vi "32 BIT ONLY  - - - - robo move.vi"() -> ()   [LabVIEW 2026]
uses:
  <vilib>/ImagingLab/Denso Robotics Library/_Private/Controls/drl_Robot Coordinates.ctl
  <vilib>/ImagingLab/Denso Robotics Library/_Private/Controls/drl_Robot Session.ctl
  <vilib>/ImagingLab/Denso Robotics Library/_Private/Controls/drl_Open Data.ctl
  <vilib>/ImagingLab/Denso Robotics Library/_Private/Controls/drl_Controller_IP Address.ctl
  <vilib>/ImagingLab/Denso Robotics Library/_Private/Controls/drl_Robot type.ctl
  <vilib>/ImagingLab/Denso Robotics Library/_Private/Controls/drl_controller_type.ctl
  <vilib>/ImagingLab/Denso Robotics Library/_Private/Controls/drl_RobSlave actions.ctl
  <vilib>/ImagingLab/Denso Robotics Library/_Private/Controls/drl_Get_Set.ctl
  <vilib>/ImagingLab/Denso Robotics Library/_Private/Controls/drl_Robot Motor status.ctl
  <vilib>/ImagingLab/Denso Robotics Library/_Private/Controls/drl_Motion parameters.ctl
  <vilib>/ImagingLab/Denso Robotics Library/_Private/Controls/drl_Interpolation.ctl
  <vilib>/ImagingLab/Denso Robotics Library/_Private/Controls/drl_Pass motion.ctl
  <vilib>/ImagingLab/Denso Robotics Library/_Private/Controls/drl_Move option.ctl
  <vilib>/ImagingLab/Denso Robotics Library/_Public/SubVIs/drl_Robot Move_CARTESIAN.vi
  <vilib>/ImagingLab/Denso Robotics Library/_Public/SubVIs/drl_Get_Robot Position_P.vi
  <vilib>/ImagingLab/Denso Robotics Library/DensoRoboticsLibrary.lvlib
panel:
  out "cRIO RT Data":cluster{u16, u16, u16}
  in  "index":i32
  out "error out":errorcluster
  in  "stop":bool
  out "Robot Position":T1 {"X" format="%.4f"; "Y" format="%.4f"; "Z" format="%.4f"; "Rx" format="%.4f"; "Ry" format="%.4f"; "Rz" format="%.4f"}
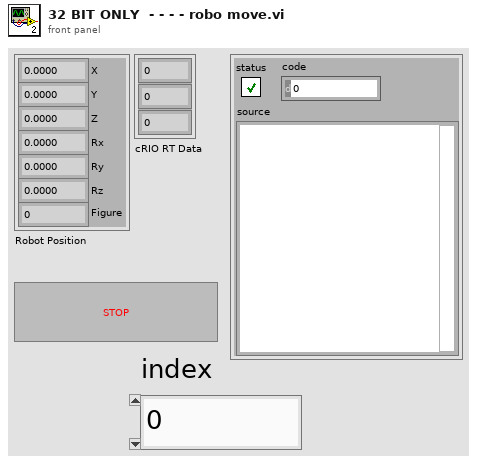
[diagram p1: front panel]
types:
  T1 = typedef "DensoRoboticsLibrary.lvlib/drl_Robot Coordinates.ctl" = cluster{"X":dbl, "Y":dbl, "Z":dbl, "Rx":dbl, "Ry":dbl, "Rz":dbl, "Figure":dbl}
  T2 = cluster{"X":dbl, "Y":dbl, "Z":dbl, "Rx":dbl, "Ry":dbl, "Rz":dbl, "Figure":dbl}
  T3 = typedef "DensoRoboticsLibrary.lvlib/drl_Motion parameters.ctl" = cluster{"Interpolation":T4, "Pass motion":T5, "Option":T6}
  T4 = typedef "DensoRoboticsLibrary.lvlib/drl_Interpolation.ctl" = enum16{"Move P", "Move L"}
  T5 = typedef "DensoRoboticsLibrary.lvlib/drl_Pass motion.ctl" = enum16{"@0", "@P", "@E"}
  T6 = typedef "DensoRoboticsLibrary.lvlib/drl_Move option.ctl" = enum16{"Default", "Next"}
  T7 = typedef "DensoRoboticsLibrary.lvlib/drl_Robot Motor status.ctl" = enum16{"Motor OFF", "Motor ON"}
  T8 = typedef "DensoRoboticsLibrary.lvlib/drl_Get_Set.ctl" = enum16{"Get", "Set"}
  T9 = typedef "DensoRoboticsLibrary.lvlib/drl_RobSlave actions.ctl" = enum16{"Start", "Stop"}
  T10 = typedef "DensoRoboticsLibrary.lvlib/drl_Open Data.ctl" = cluster{"controller IP address":T11, "robot type":T12, "controller type":T13}
  T11 = typedef "DensoRoboticsLibrary.lvlib/drl_Controller_IP Address.ctl" = string
  T12 = typedef "DensoRoboticsLibrary.lvlib/drl_Robot type.ctl" = enum16{"6 axes", "5 axes", "4 axes"}
  T13 = typedef "DensoRoboticsLibrary.lvlib/drl_controller_type.ctl" = enum16{"RC7", "RC8"}
  T14 = typedef "DensoRoboticsLibrary.lvlib/drl_Robot Session.ctl" = string
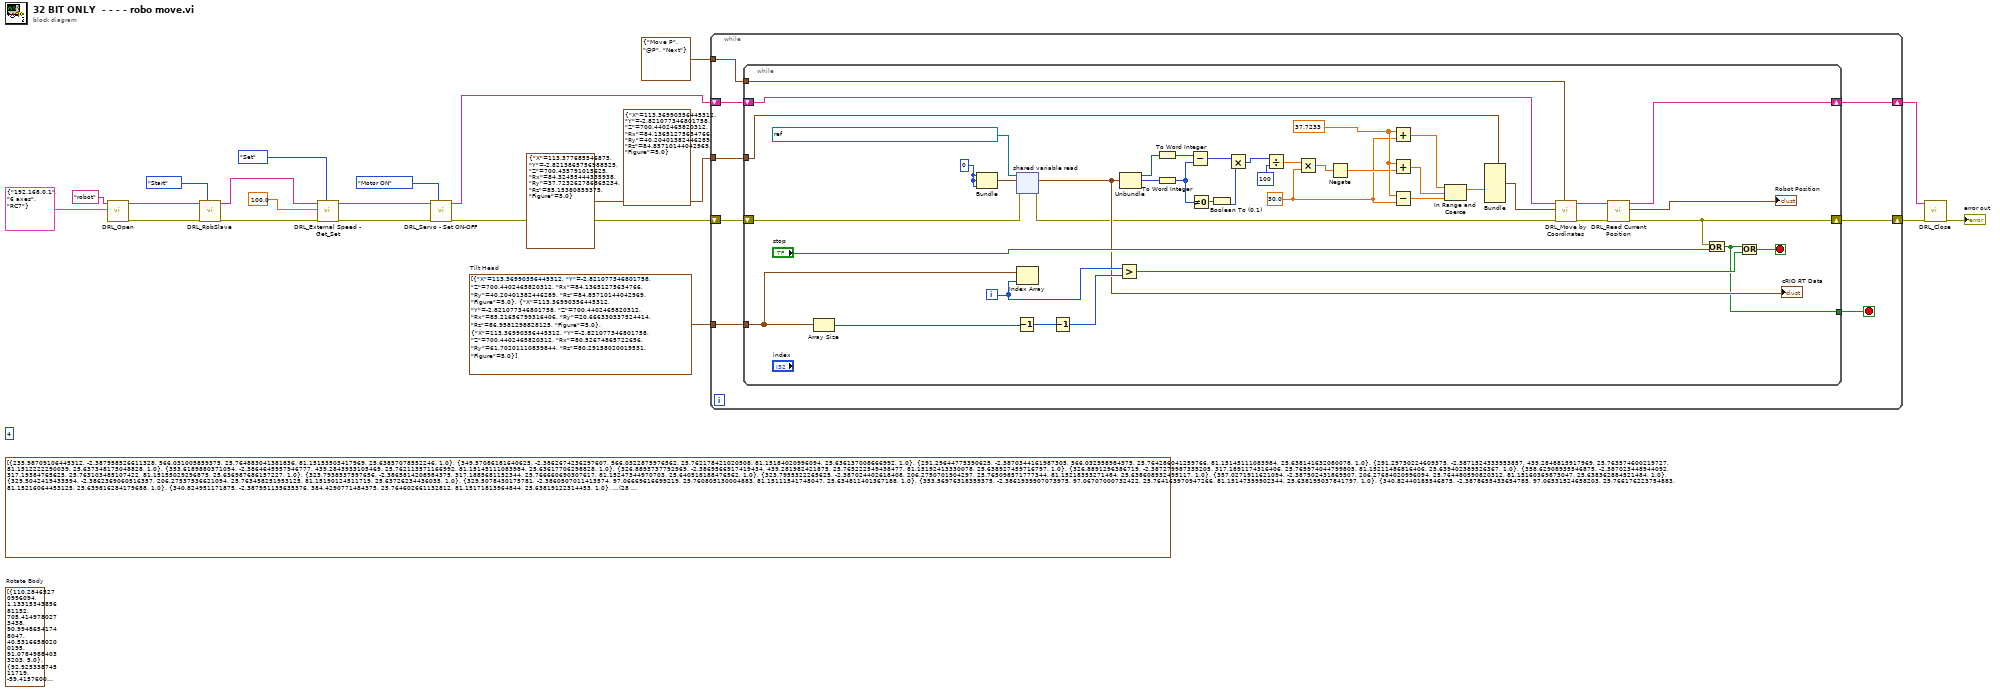
[diagram p0: block diagram]
diagram:
  (unwired) T1 {"X"=113.36990356445312, "Y"=-2.821077346801758, "Z"=700.4402465820312, "Rx"=84.13651275634766, "Ry"=40.20401382446289, "Rz"=84.85710144042969, "Figure"=5.0} ("position P")
  w2 = T1[] [{"X"=113.36990356445312, "Y"=-2.821077346801758, "Z"=700.4402465820312, "Rx"=84.13651275634766, "Ry"=40.20401382446289, "Rz"=84.85710144042969, "Figure"=5.0}, {"X"=113.36990356445312, "Y"=-2.821077346801758, "Z"=700.4402465820312, "Rx"=85.21656799316406, "Ry"=20.666330337524414, "Rz"=86.9581298828125, "Figure"=5.0}, {"X"=113.36990356445312, "Y"=-2.821077346801758, "Z"=700.4402465820312, "Rx"=80.52674865722656, "Ry"=61.70201110839844, "Rz"=80.29158020019531, "Figure"=5.0}]  # Tilt Head
  (unwired) T1[] [{"X"=110.28465270996094, "Y"=1.1331534385681152, "Z"=705.4149780273438, "Rx"=90.99486541748047, "Ry"=40.53166580200195, "Rz"=91.07849884033203, "Figure"=5.0}, {"X"=92.92533874511719, "Y"=-59.4157600402832, "Z"=705.412109375, "Rx"=90.99667358398438, "Ry"=40.53141784667969, "Rz"=57.89656448364258, "Figure"=5.0}, {"X"=90.63916778564453, "Y"=62.848175048828125, "Z"=705.412109375, "Rx"=90.99667358398438, "Ry"=40.53141784667969, "Rz"=125.22810363769531, "Figure"=5.0}]  # Rotate Body
  (unwired) T1[] [{"X"=235.98709106445312, "Y"=-2.387958526611328, "Z"=566.031005859375, "Rx"=25.764883041381836, "Ry"=81.15153503417969, "Rz"=25.63857078552246, "Figure"=1.0}, {"X"=349.57086181640625, "Y"=-2.3862674236297607, "Z"=566.0322875976562, "Rx"=25.762178421020508, "Ry"=81.15184020996094, "Rz"=25.636137008666992, "Figure"=1.0}, {"X"=291.29644775390625, "Y"=-2.3870344161987305, "Z"=566.032958984375, "Rx"=25.764286041259766, "Ry"=81.15145111083984, "Rz"=25.638141632080078, "Figure"=1.0}, {"X"=291.29730224609375, "Y"=-2.3871524333953857, "Z"=439.2848815917969, "Rx"=25.763574600219727, "Ry"=81.1512222290039, "Rz"=25.637348175048828, "Figure"=1.0}, {"X"=353.6189880371094, "Y"=-2.3864645957946777, "Z"=439.2843933105469, "Rx"=25.762113571166992, "Ry"=81.15145111083984, "Rz"=25.63617706298828, "Figure"=1.0}, {"X"=326.8893737792969, "Y"=-2.3869566917419434, "Z"=439.281982421875, "Rx"=25.765222549438477, "Ry"=81.15192413330078, "Rz"=25.638927459716797, "Figure"=1.0}, {"X"=326.8891296386719, "Y"=-2.387279987335205, "Z"=317.1891174316406, "Rx"=25.765974044799805, "Ry"=81.15211486816406, "Rz"=25.639402389526367, "Figure"=1.0}, {"X"=358.62908935546875, "Y"=-2.387023448944092, "Z"=317.19384765625, "Rx"=25.763103485107422, "Ry"=81.15155029296875, "Rz"=25.636987686157227, "Figure"=1.0}, {"X"=323.7938537597656, "Y"=-2.3865814208984375, "Z"=317.1885681152344, "Rx"=25.766660690307617, "Ry"=81.15247344970703, "Rz"=25.640518188476562, "Figure"=1.0}, {"X"=323.7955322265625, "Y"=-2.387024402618408, "Z"=206.2750701904297, "Rx"=25.765098571777344, "Ry"=81.15218353271484, "Rz"=25.638608932495117, "Figure"=1.0}, {"X"=357.0271911621094, "Y"=-2.387502431869507, "Z"=206.27684020996094, "Rx"=25.764480590820312, "Ry"=81.15160369873047, "Rz"=25.638362884521484, "Figure"=1.0}, {"X"=329.5042419433594, "Y"=-2.3862369060516357, "Z"=206.27537536621094, "Rx"=25.763458251953125, "Ry"=81.15190124511719, "Rz"=25.63726234436035, "Figure"=1.0}, {"X"=329.5078430175781, "Y"=-2.3860507011413574, "Z"=97.06669616699219, "Rx"=25.760805130004883, "Ry"=81.15111541748047, "Rz"=25.634811401367188, "Figure"=1.0}, {"X"=353.56976318359375, "Y"=-2.3861939907073975, "Z"=97.06707000732422, "Rx"=25.764163970947266, "Ry"=81.15147399902344, "Rz"=25.638195037841797, "Figure"=1.0}, {"X"=340.82440185546875, "Y"=-2.3878655433654785, "Z"=97.06531524658203, "Rx"=25.766176223754883, "Ry"=81.15216064453125, "Rz"=25.639816284179688, "Figure"=1.0}, {"X"=340.824951171875, "Y"=-2.387951135635376, "Z"=384.4290771484375, "Rx"=25.764602661132812, "Ry"=81.15171813964844, "Rz"=25.63819122314453, "Figure"=1.0}, {"X"=1.4659475088119507, "Y"=-340.9820861816406, "Z"=384.4298400878906, "Rx"=25.765399932861328, "Ry"=81.15129089355469, "Rz"=-63.7135124206543, "Figure"=1.0}, {"X"=1.4659475088119507, "Y"=-340.9820861816406, "Z"=384.4298400878906, "Rx"=25.765399932861328, "Ry"=81.15129089355469, "Rz"=-63.7135124206543, "Figure"=1.0}, {"X"=1.4495900869369507, "Y"=-336.9073791503906, "Z"=400.07806396484375, "Rx"=9.859703063964844, "Ry"=68.43805694580078, "Rz"=-79.16173553466797, "Figure"=1.0}, {"X"=1.449590802192688, "Y"=-336.9075927734375, "Z"=400.07757568359375, "Rx"=9.859916687011719, "Ry"=68.43849182128906, "Rz"=-79.16153717041016, "Figure"=1.0}, {"X"=1.4632148742675781, "Y"=-340.8019714355469, "Z"=363.8247375488281, "Rx"=156.8294677734375, "Ry"=80.24137878417969, "Rz"=66.77577209472656, "Figure"=1.0}, {"X"=1.4495900869369507, "Y"=-336.9073791503906, "Z"=400.07806396484375, "Rx"=9.859703063964844, "Ry"=68.43805694580078, "Rz"=-79.16173553466797, "Figure"=1.0}, {"X"=1.4632148742675781, "Y"=-340.8019714355469, "Z"=363.8247375488281, "Rx"=156.8294677734375, "Ry"=80.24137878417969, "Rz"=66.77577209472656, "Figure"=1.0}, {"X"=1.4669764041900635, "Y"=-341.2671813964844, "Z"=382.1100769042969, "Rx"=32.499534606933594, "Ry"=82.82139587402344, "Rz"=-57.044464111328125, "Figure"=1.0}, {"X"=340.9021301269531, "Y"=-15.848700523376465, "Z"=382.1100769042969, "Rx"=32.49953079223633, "Ry"=82.82139587402344, "Rz"=30.047452926635742, "Figure"=1.0}, {"X"=340.9021301269531, "Y"=-15.848700523376465, "Z"=382.1100769042969, "Rx"=32.49953079223633, "Ry"=82.82139587402344, "Rz"=30.047452926635742, "Figure"=1.0}, {"X"=340.9021301269531, "Y"=-15.848700523376465, "Z"=382.1100769042969, "Rx"=32.49953079223633, "Ry"=82.82139587402344, "Rz"=30.047452926635742, "Figure"=1.0}, {"X"=340.9021301269531, "Y"=-15.848700523376465, "Z"=382.1100769042969, "Rx"=32.49953079223633, "Ry"=82.82139587402344, "Rz"=30.047452926635742, "Figure"=1.0}] ("appended array")
  (unwired) 4
  n1 = call <vilib>:"DRL_Open.vi"("connection settings"=T10 {"controller IP address"="192.168.0.1", "robot type"=enum."6 axes", "controller type"=enum."RC7"}, "robot session"=T14 "robot") -> ("error out"=w6:errorcluster, "robot session*"=w7:T14)  [unwired: 8 in]
  n2 = call <vilib>:"DRL_RobSlave.vi"("action"=drl_RobSlave_actions."Start" ("Action"), "error in (no error)"=w6, "robot session"=w7) -> ("error out"=w8:errorcluster, "robot session*"=w9:T14)  [unwired: 7 out]
  n3 = call <vilib>:"DRL_External Speed - Get_Set.vi"("action"=drl_Get_Set."Set" ("Get / Set"), "error in (no error)"=w8, "ext speed in"=sgl 100.0 ("Ext Speed in"), "robot session"=w9) -> ("error out"=w11:errorcluster, "robot session*"=w10:T14)  [unwired: 6 out]
  n4 = call <vilib>:"DRL_Servo - Set ON-OFF.vi"("servo status"=drl_Robot_Motor_status."Motor ON" ("Motor Status"), "error in (no error)"=w11, "robot session"=w10) -> ("error out"=w4:errorcluster, "robot session*"=w5:T14)  [unwired: 7 out]
  n5 = while {
    tunnel: T3 {"Interpolation"=enum."Move P", "Pass motion"=enum."@P", "Option"=enum."Next"} ("motion parameters") -> [w24]
    shift-right: [w27] -> w17
    shift-left: w5 -> [w26]
    shift-right: [w28] -> w18
    shift-left: w4 -> [w25]
    tunnel: w2 -> [w23]
    tunnel: T2 {"X"=113.377685546875, "Y"=-2.8213865756988525, "Z"=700.435791015625, "Rx"=84.32455444335938, "Ry"=37.723262786865234, "Rz"=85.15380859375, "Figure"=5.0} -> [w21]
    stop <- w22 stop-if-true
    n6 = while {
      shift-right: [w68] -> w28
      shift-left: w25 -> [w30]
      shift-right: [w70] -> w27
      shift-left: w26 -> [w67]
      tunnel: w24 -> [w64]
      tunnel: w23 -> [w57]
      tunnel: [w35] -> w22
      tunnel: w21 -> [w55]
      i -> [w63]
      stop <- w61 stop-if-true
      w40 = 37.7233 ("y")
      w38 = 30.0 ("y")
      w52 = u16 0
      n7 = Array Size(array=w57) -> (size(s)=w62:i32)
      n8 = Bundle(w52, w52, w52) -> (w53:cluster{u16, u16, u16})  [unwired: 1 in]
      n9 = Decrement(x=w62) -> (x-1=w58:i32)
      n10 = shared-variable-read(refnum<k21> "ni.var.psp://SpeedOfVIght/RT ShardVariables/Final Score" ("shared variable refnum in"), w30, w53) -> (w29:errorcluster, w50:cluster{u16, u16, u16})  [unwired: 2 out]
      "cRIO RT Data" <- w50
      n11 = Index Array(array=w57, index=w63) -> ()  [unwired: 1 out]
      n12 = Decrement(x=w58) -> (x-1=w59:i32)
      n13 = Greater?(x=w63, y=w59) -> (0:w60:bool)
      n14 = Unbundle(w50) -> (w49:u16, w48:u16)  [unwired: 1 out]
      n15 = To Word Integer(number=w49) -> (16bit integer=w41:i16)
      n16 = To Word Integer(number=w48) -> (16bit integer=w34:i16)
      n17 = Subtract(x=w41, y=w34) -> (x-y=w47:i16)
      n18 = Not Equal To 0?(x=w34) -> (x != 0?=w33:bool)
      n19 = Boolean To (0,1)(Boolean=w33) -> (0, 1=w31:i16)
      n20 = Multiply(x=w47, y=w31) -> (x*y=w32:i16)
      n21 = Divide(x=w32, y=u16 100) -> (x/y=w45:dbl)
      n22 = Multiply(x=w45, y=w38) -> (x*y=w44:dbl)
      n23 = Negate(x=w44) -> (-x=w39:dbl)
      n24 = Add(x=w40, y=w38) -> (x+y=w37:dbl)
      n25 = Add(x=w40, y=w39) -> (x+y=w43:dbl)
      n26 = Subtract(x=w40, y=w38) -> (x-y=w36:dbl)
      n27 = In Range and Coerce(upper limit=w37, x=w43, lower limit=w36) -> (coerced(x)=w54:dbl)  [unwired: 1 out]
      n28 = Bundle(cluster=w55, "Ry"=w54) -> (w42:T2)  [unwired: 6 in]
      n29 = call-poly <vilib>:"DRL_Move by Coordinates.vi"("motion parameters"=w64, "error in (no error)"=w29, "robot coordinates"=w42, "robot session"=w67) -> ("error out"=w66:errorcluster, "robot session*"=w65:T14)  [unwired: 6 out]
      n30 = call-poly <vilib>:"DRL_Read Current Position.vi"("error in (no error)"=w66, "robot session"=w65) -> ("error out"=w68:errorcluster, "position P"=→"Robot Position":T1, "robot session*"=w70:T14)  [unwired: 7 in]
      n31 = Or(x=w68, y="stop") -> (x .or. y?=w35:bool)
      n32 = Or(x=w35, y=w60) -> (x .or. y?=w61:bool)
    }
  }
  n33 = call <vilib>:"DRL_Close.vi"("error in (no error)"=w18, "robot session"=w17) -> ("error out"=→"error out":errorcluster)  [unwired: 9 in]
